vi "DHE_GetCallback.vi"() -> (7 "DHE_CallBack":T1)   [LabVIEW 2016]
uses:
  private/vis/DHE_GBLDriverVariables.vi
  Common/public/vis/SCL_Pending Action.ctl
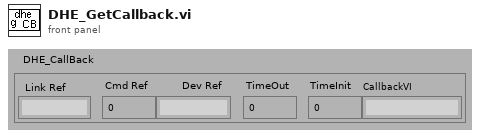
[diagram p1: front panel]
types:
  T1 = typedef "SCL_Pending Action.ctl" = cluster{"Cmd Ref":i32, "Dev Ref":string, "TimeOut":i32, "TimeInit":i32, "CallbackVI":string, "Link Ref":string}
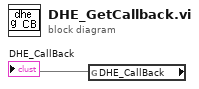
[diagram p0: block diagram]
diagram:
  n1 = global read "DHE_GBLDriverVariables.vi" "DHE_CallBack"() -> (→"DHE_CallBack")
